vi "WLAN - niVST - RFSG - Select Wfm and Set IQ Rate.vi"(0 "instrument handle":refnum<k15>, 1 "Wfm Name":string, 11 "error in":errorcluster, 12 "Wfm Index":i32, 13 "dt":dbl) -> (4 "instrument handle":refnum<k15>, 15 "error out":errorcluster)   [LabVIEW 2011]
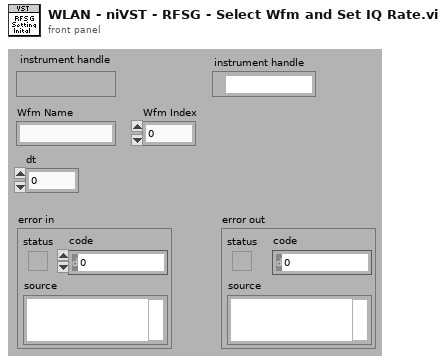
[diagram p1: front panel]
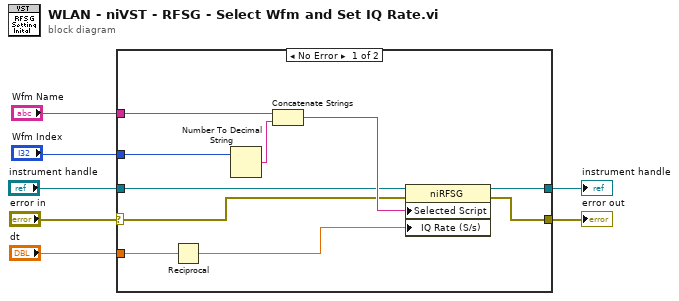
[diagram p0: block diagram]
diagram:
  n1 = case shown="No Error" "error in" {
    selector: "error in" -> [w14 w18]
    tunnel: [w13 w18] -> w6
    tunnel: "instrument handle" -> [w12 w19]
    tunnel: [w11 w19] -> w4
    tunnel: "dt" -> [w10 _]
    tunnel: "Wfm Index" -> [w9 _]
    tunnel: "Wfm Name" -> [w8 _]
    frame No Error {
      n2 = Reciprocal(x=w10) -> (1/x=w15:dbl)
      n3 = Number To Decimal String(number=w9) -> (decimal integer string=w17:string)  [unwired: 1 in]
      n4 = Concatenate Strings(w8, w17) -> (w16:string)
      n5 = property class="niRFSG"(reference=w12, error in=w14, "Selected Script"=w16, "IQ Rate (S/s)"=w15) -> (reference out=w11:refnum<k15>, error out=w13:errorcluster)
    }
    frame Error {
    }
  }
  "error out" <- w6
  "instrument handle" <- w4
